vi "Heart Rate Simulator.vi"() -> ()   [LabVIEW 2018, in "Heart Rate Simulator.lvlib"]
uses:
  Heart Rate Simulator.lvlib
  Program Files (x86)/National Instruments/LabVIEW 2018/examples/Instrument IO/Serial/support/Serial - Settings.ctl
  Program Files (x86)/National Instruments/LabVIEW 2018/examples/Instrument IO/Serial/support/Serial - XON-XOFF Characters.ctl
  Program Files (x86)/National Instruments/LabVIEW 2018/examples/Instrument IO/Serial/support/Serial - ASCII Characters.ctl
  <vilib>/Instr/_visa.llb/VISA Configure Serial Port (Instr).vi
panel:
  in  "Stop":bool
  in  "Termination Character":u8=10 format="%.0x"
  in  "End Write on Termination Character?":bool=TRUE
  in  "XON/XOFF Characters":T1={"XON"=enum."DC1", "XOFF"=enum."DC3"}
  in  "Serial Settings":T3={"baud rate"=9600, "data bits"=8, "parity"=enum."None", "stop bits"=10, "flow control"=0} {"flow control" items=["None"=0, "XON/XOFF"=1, "RTS/CTS"=2, "DTR/DSR"=4]; "stop bits" items=["1.0"=10, "1.5"=15, "2.0"=20]; "data bits" min=5 max=8 step=1; "baud rate" items=["75"=75, "110"=110, "134"=134, "150"=150, "300"=300, "600"=600, "1200"=1200, "1800"=1800, "2400"=2400, "4800"=4800, "7200"=7200, "9600"=9600, "14400"=14400, "19200"=19200, "28800"=28800, "38400"=38400, "56000"=56000, "57600"=57600, "115200"=115200, "128000"=128000, "230400"=230400]}
  in  "VISA resource name":refnum<visa-resource-name>="COM1"
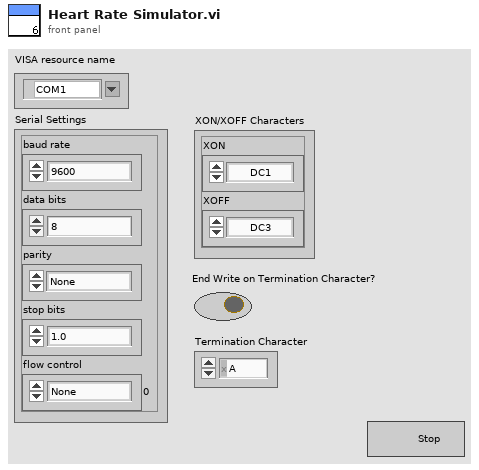
[diagram p1: front panel]
types:
  T1 = typedef "Serial - XON-XOFF Characters.ctl" = cluster{"XON":T2, "XOFF":T2}
  T2 = typedef "Serial - ASCII Characters.ctl" = enum16{"NUL", "SOH", "STX", "ETX", "EOT", "ENQ", "ACK", "BEL", "BS", "HT", "LF", "VT", "FF", "CR", "SO", "SI", "DLE", "DC1", "DC2", "DC3", "DC4", "NAK", "SYN", "ETB", "CAN", "EM", "SUB", "ESC", "FS", "GS", "RS", "US", "SP", "!", "\"", "#", "$", "%", "&", "'", "(", ")", "*", "+", ",", "- (-)", ".", "/", "0", "1", "2", "3", "4", "5", "6", "7", "8", "9", ":", ";", "<", "=", ">", "?", "@", "A", "B", "C", "D", "E", "F", "G", "H", "I", "J", "K", "L", "M", "N", "O", "P", "Q", "R", "S", "T", "U", "V", "W", "X", "Y", "Z", "[", "\\", "]", "^", "_", "`", "a", "b", "c", "d", "e", "f", "g", "h", "i", "j", "k", "l", "m", "n", "o", "p", "q", "r", "s", "t", "u", "v", "w", "x", "y", "z", "{", "|", "}", "~"}
  T3 = typedef "Serial - Settings.ctl" = cluster{"baud rate":u32, "data bits":u16, "parity":enum16{"None", "Odd", "Even", "Mark", "Space"}, "stop bits":u16, "flow control":u16}
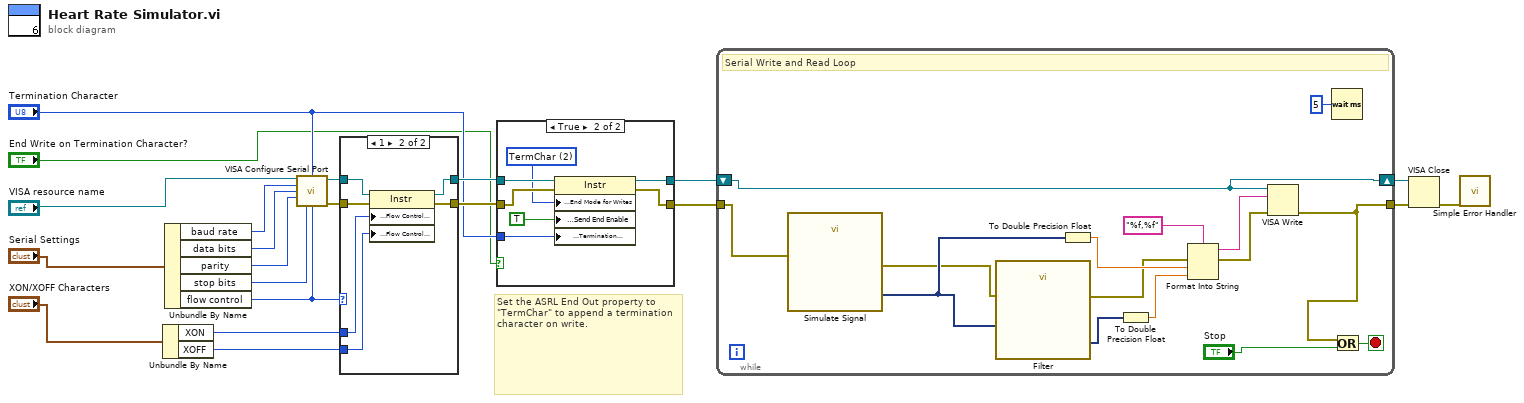
[diagram p0: block diagram]
diagram:
  # "Set the ASRL End Out property to \"TermChar\" to append a termination character on write."
  n1 = Unbundle By Name("XON/XOFF Characters") -> ("XON"=w14:T2, "XOFF"=w13:T2)
  n2 = Unbundle By Name("Serial Settings") -> ("baud rate"=w16:u32, "data bits"=w17:u16, "parity"=w18:enum16{"None", "Odd", "Even", "Mark", "Space"}, "stop bits"=w19:u16, "flow control"=w15:u16)
  n3 = call-poly "VISA Configure Serial Port"("VISA resource name"="VISA resource name", "termination char\n(0xA = '\\n' = LF)"="Termination Character", "baud rate (9600)"=w16, "data bits (8)"=w17, "parity (0:none)"=w18, "stop bits (10: 1 bit)"=w19, "flow control (0:none)"=w15) -> ("VISA resource name out"=w20:refnum<visa-resource-name>, "error out"=w21:errorcluster)  [unwired: 3 in, 4 out]
  n4 = case shown="1" w15 {
    tunnel: [w22 w29] -> w5
    tunnel: [w23 w28] -> w6
    tunnel: w21 -> [w22 w27]
    tunnel: w20 -> [w23 w26]
    tunnel: w14 -> [_ w25]
    tunnel: w13 -> [_ w24]
    frame Default {
    }
    frame 1 {
      n5 = property class="Instr"(reference=w26, error in=w27, "Serial Settings:Flow Control XON Character"=w25, "Serial Settings:Flow Control XOFF Character"=w24) -> (reference out=w28:refnum<visa-resource-name>, error out=w29:errorcluster)
    }
  }
  n6 = case shown="True" "End Write on Termination Character?" {
    tunnel: w6 -> [w30 w38]
    tunnel: w5 -> [w31 w37]
    tunnel: [w30 w36] -> w3
    tunnel: [w31 w35] -> w2
    tunnel: "Termination Character" -> [_ w33]
    frame False {
    }
    frame True {
      w34 = u16 2 items=["None", "LastBit", "TermChar", "Break"] ("Serial Settings:Serial End Mode for Writes")
      n7 = property class="Instr"(reference=w38, error in=w37, "Serial Settings:End Mode for Writes"=w34, "Message Based Settings:Send End Enable"=TRUE, "Message Based Settings:Termination Character"=w33) -> (reference out=w36:refnum<visa-resource-name>, error out=w35:errorcluster)
    }
  }
  n8 = while {
    shift-right: [w44] -> w8
    shift-left: w3 -> [w44]
    tunnel: w2 -> [w42]
    tunnel: [w50] -> w9
    stop <- w52 stop-if-true
    # "Serial Write and Read Loop"
    n9 = call "Simulate Signal"("error in (no error)"=w42) -> ("Sine"=w48:dynamicdata, "error out"=w41:errorcluster)  [unwired: 13 in]
    n10 = call "Filter"("error in (no error)"=w41, "Signal"=w48) -> ("error out"=w40:errorcluster, "Filtered Signal"=w46:dynamicdata)  [unwired: 8 in]
    n11 = To Double Precision Float(number=w48) -> (double precision float=w47:dbl)
    n12 = To Double Precision Float(number=w46) -> (double precision float=w45:dbl)
    n13 = Format Into String(format string="%f,%f", error in=w40, w47, w45) -> (resulting string=w43:string, error out=w39:errorcluster)  [unwired: 1 in]
    n14 = VISA Write(VISA resource name=w44, write buffer=w43, error in (no error)=w39) -> (error out=w50:errorcluster)  [unwired: 2 out]
    n15 = Wait (ms)(milliseconds to wait=u32 5) -> ()  [unwired: 1 out]
    n16 = Or(x=w50, y="Stop") -> (x .or. y?=w52:bool)
  }
  n17 = VISA Close(VISA resource name=w8, error in (no error)=w9) -> (error out=w7:errorcluster)
  n18 = call <vilib>:"Simple Error Handler.vi"("error in (no error)"=w7) -> ()  [unwired: 1 in, 8 out]
